vi "Add session file to index.vi"(6 "Workspace path":path, 7 "User":string, 8 "error in (no error)":errorcluster, 9 "ZIP file path":path, 10 "Session name":string, 11 "Index File Path":path) -> (0 "error out":errorcluster, 3 "Index":T1[](array[typedef]))   [LabVIEW 2019]
doc: "Adds a session file to index of oppened files"
uses:
  Type defs/Opened session file info Type Def.ctl
  Type defs/Opened session file index Type Def.ctl
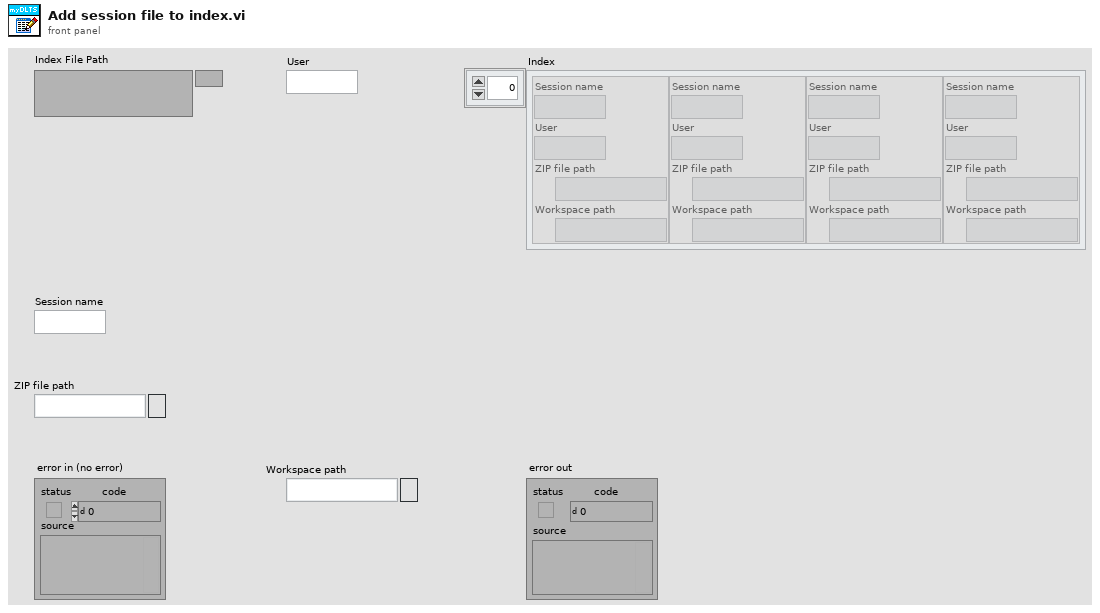
[diagram p1: front panel]
types:
  T1 = typedef "Opened session file info Type Def.ctl" = cluster{"Session name":string, "User":string, "ZIP file path":path, "Workspace path":path}
  T2 = typedef "Opened session file index Type Def.ctl" = cluster{"File":T1[]}
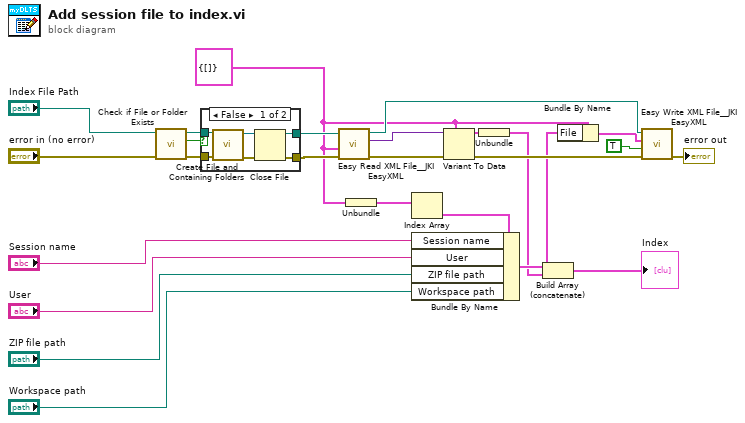
[diagram p0: block diagram]
diagram:
  w3 = T2 {"File"=[]} ("Index")
  n1 = call <vilib>:"Check if File or Folder Exists.vi"("error in (no error)"="error in (no error)", "path"="Index File Path") -> ("error out"=w12:errorcluster, "file or folder exists?"=w10:bool, "dup path"=w11:path)  [unwired: 7 in]
  n2 = case shown="False" w10 {
    tunnel: w12 -> [w31 w32]
    tunnel: w11 -> [w30 w33]
    tunnel: [w27 w33] -> w8
    tunnel: [w26 w32] -> w9
    frame False {
      n3 = call <vilib>:"Create File and Containing Folders.vi"("error in (no error)"=w31, "file path"=w30) -> ("error out"=w29:errorcluster, "refnum out"=w28:refnum<file>)  [unwired: 8 in]
      n4 = Close File(refnum=w28, error in=w29) -> (path=w27:path, error out=w26:errorcluster)
    }
    frame True {
    }
  }
  n5 = call <vilib>:"Easy Read XML File__JKI EasyXML.vi"("error in (no error)"=w9, "LabVIEW Data (Type)"=w3, "XML File Path"=w8) -> ("error out"=w25:errorcluster, "LabVIEW Data"=w22:variant, "XML File Path (duplicate)"=w21:path)  [unwired: 6 in]
  n6 = Unbundle(w3) -> ("File"=w5:T1[])
  n7 = Index Array(array=w5) -> (element=w19:T1)  [unwired: 1 in]
  n8 = Bundle By Name(cluster=w19, "Session name"="Session name", "User"="User", "ZIP file path"="ZIP file path", "Workspace path"="Workspace path") -> (w18:T1)
  n9 = Variant To Data(error in=w25, type=w3, Variant=w22) -> (data=w20:T2, error out=w24:errorcluster)
  n10 = Unbundle(w20) -> ("File"=w4:T1[])
  n11 = Build Array (concatenate)(w18, w4) -> (w2:T1[])
  "Index" <- w2
  n12 = Bundle By Name(cluster=w3, "File"=w2) -> (w1:T2)
  n13 = call <vilib>:"Easy Write XML File__JKI EasyXML.vi"("error in (no error)"=w24, "Overwrite File? (false)"=TRUE, "LabVIEW Data"=w1, "XML File Path"=w21) -> ("error out"=→"error out":errorcluster)  [unwired: 6 in, 1 out]
